vi "Unit test on Decode response.vi"() -> (0 "Error array":errorcluster[](array[cluster]), 2 "Test results":T1(array[cluster]), 3 "Passed":bool)   [LabVIEW 2021, in "F-70 driver.lvlib"]
uses:
  F-70 driver.lvlib
  public/F-70 parameters.ctl
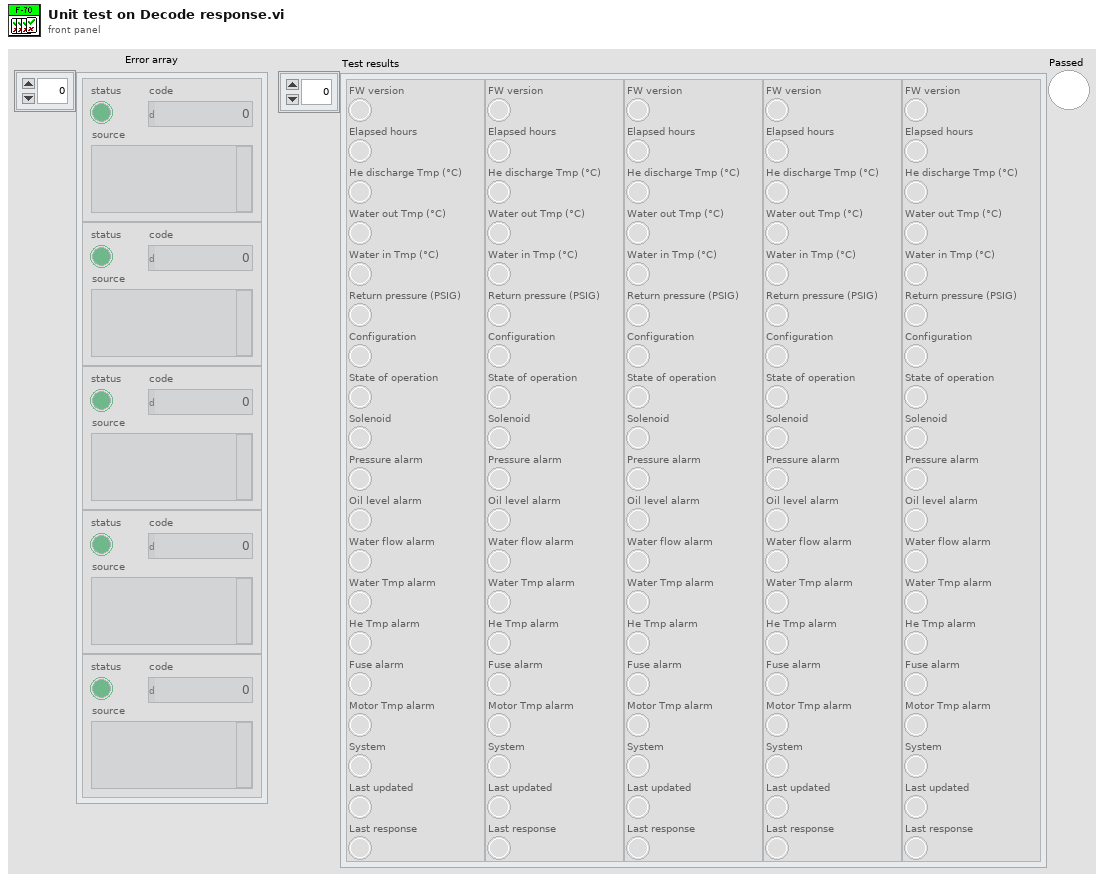
[diagram p1: front panel]
types:
  T1 = cluster{"FW version":bool, "Elapsed hours":bool, "He discharge Tmp (°C)":bool, "Water out Tmp (°C)":bool, "Water in Tmp (°C)":bool, "Return pressure (PSIG)":bool, "Configuration":bool, "State of operation":bool, "Solenoid":bool, "Pressure alarm":bool, "Oil level alarm":bool, "Water flow alarm":bool, "Water Tmp alarm":bool, "He Tmp alarm":bool, "Fuse alarm":bool, "Motor Tmp alarm":bool, "System":bool, "Last updated":bool, "Last response":bool}[]
  T2 = typedef "F-70 driver.lvlib/F-70 parameters.ctl" = cluster{"FW version":dbl, "Elapsed hours":dbl, "He discharge Tmp (°C)":dbl, "Water out Tmp (°C)":dbl, "Water in Tmp (°C)":dbl, "Return pressure (PSIG)":dbl, "Configuration":bool, "State of operation":u16, "Solenoid":bool, "Pressure alarm":bool, "Oil level alarm":bool, "Water flow alarm":bool, "Water Tmp alarm":bool, "He Tmp alarm":bool, "Fuse alarm":bool, "Motor Tmp alarm":bool, "System":bool, "Last updated":timestamp, "Last response":string}
  T3 = cluster{"FW version":bool, "Elapsed hours":bool, "He discharge Tmp (°C)":bool, "Water out Tmp (°C)":bool, "Water in Tmp (°C)":bool, "Return pressure (PSIG)":bool, "Configuration":bool, "State of operation":bool, "Solenoid":bool, "Pressure alarm":bool, "Oil level alarm":bool, "Water flow alarm":bool, "Water Tmp alarm":bool, "He Tmp alarm":bool, "Fuse alarm":bool, "Motor Tmp alarm":bool, "System":bool, "Last updated":bool, "Last response":bool}
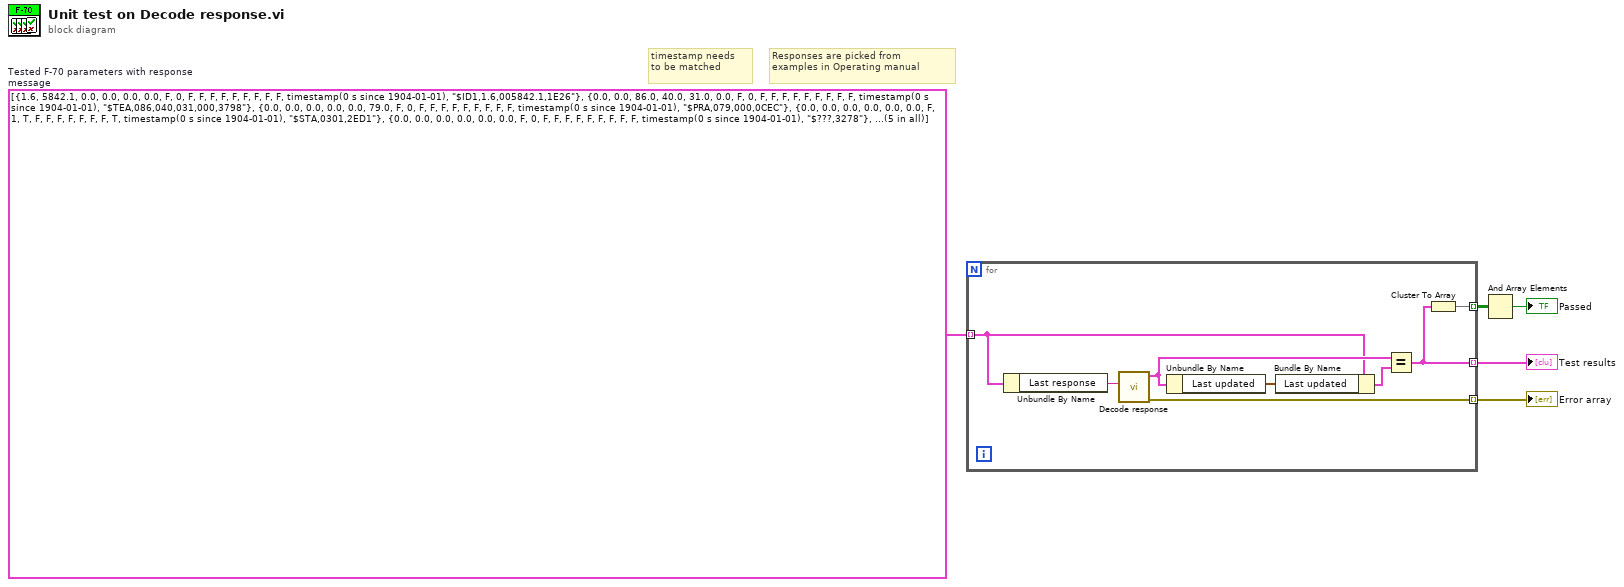
[diagram p0: block diagram]
diagram:
  w5 = T2[] [{"FW version"=1.6, "Elapsed hours"=5842.1, "He discharge Tmp (°C)"=0.0, "Water out Tmp (°C)"=0.0, "Water in Tmp (°C)"=0.0, "Return pressure (PSIG)"=0.0, "Configuration"=FALSE, "State of operation"=0, "Solenoid"=FALSE, "Pressure alarm"=FALSE, "Oil level alarm"=FALSE, "Water flow alarm"=FALSE, "Water Tmp alarm"=FALSE, "He Tmp alarm"=FALSE, "Fuse alarm"=FALSE, "Motor Tmp alarm"=FALSE, "System"=FALSE, "Last updated"=timestamp(0 s since 1904-01-01), "Last response"="$ID1,1.6,005842.1,1E26"}, {"FW version"=0.0, "Elapsed hours"=0.0, "He discharge Tmp (°C)"=86.0, "Water out Tmp (°C)"=40.0, "Water in Tmp (°C)"=31.0, "Return pressure (PSIG)"=0.0, "Configuration"=FALSE, "State of operation"=0, "Solenoid"=FALSE, "Pressure alarm"=FALSE, "Oil level alarm"=FALSE, "Water flow alarm"=FALSE, "Water Tmp alarm"=FALSE, "He Tmp alarm"=FALSE, "Fuse alarm"=FALSE, "Motor Tmp alarm"=FALSE, "System"=FALSE, "Last updated"=timestamp(0 s since 1904-01-01), "Last response"="$TEA,086,040,031,000,3798"}, {"FW version"=0.0, "Elapsed hours"=0.0, "He discharge Tmp (°C)"=0.0, "Water out Tmp (°C)"=0.0, "Water in Tmp (°C)"=0.0, "Return pressure (PSIG)"=79.0, "Configuration"=FALSE, "State of operation"=0, "Solenoid"=FALSE, "Pressure alarm"=FALSE, "Oil level alarm"=FALSE, "Water flow alarm"=FALSE, "Water Tmp alarm"=FALSE, "He Tmp alarm"=FALSE, "Fuse alarm"=FALSE, "Motor Tmp alarm"=FALSE, "System"=FALSE, "Last updated"=timestamp(0 s since 1904-01-01), "Last response"="$PRA,079,000,0CEC"}, {"FW version"=0.0, "Elapsed hours"=0.0, "He discharge Tmp (°C)"=0.0, "Water out Tmp (°C)"=0.0, "Water in Tmp (°C)"=0.0, "Return pressure (PSIG)"=0.0, "Configuration"=FALSE, "State of operation"=1, "Solenoid"=TRUE, "Pressure alarm"=FALSE, "Oil level alarm"=FALSE, "Water flow alarm"=FALSE, "Water Tmp alarm"=FALSE, "He Tmp alarm"=FALSE, "Fuse alarm"=FALSE, "Motor Tmp alarm"=FALSE, "System"=TRUE, "Last updated"=timestamp(0 s since 1904-01-01), "Last response"="$STA,0301,2ED1"}, {"FW version"=0.0, "Elapsed hours"=0.0, "He discharge Tmp (°C)"=0.0, "Water out Tmp (°C)"=0.0, "Water in Tmp (°C)"=0.0, "Return pressure (PSIG)"=0.0, "Configuration"=FALSE, "State of operation"=0, "Solenoid"=FALSE, "Pressure alarm"=FALSE, "Oil level alarm"=FALSE, "Water flow alarm"=FALSE, "Water Tmp alarm"=FALSE, "He Tmp alarm"=FALSE, "Fuse alarm"=FALSE, "Motor Tmp alarm"=FALSE, "System"=FALSE, "Last updated"=timestamp(0 s since 1904-01-01), "Last response"="$???,3278"}]  # Tested F-70 parameters with response message
  # "Responses are picked from \nexamples in Operating manual"
  # "timestamp needs\nto be matched"
  n1 = for {
    tunnel: w5 -> [w6] mode=indexing
    tunnel: [w13] -> w4 mode=indexing
    tunnel: [w11] -> w3 mode=indexing
    tunnel: [w10] -> w2 mode=indexing
    n2 = Unbundle By Name(w6) -> ("Last response"=w12:string)
    n3 = call "Decode response.vi"("response in"=w12) -> ("error out"=w13:errorcluster, "F-70 parameters out"=w7:T2)  [unwired: 9 in]
    n4 = Unbundle By Name(w7) -> ("Last updated"=w9:timestamp)
    n5 = Bundle By Name(cluster=w6, "Last updated"=w9) -> (w8:T2)
    n6 = Equal?(x=w7, y=w8) -> (x = y?=w11:T3)
    n7 = Cluster To Array(cluster=w11) -> (array=w10:bool[])
  }
  "Error array" <- w4
  "Test results" <- w3
  n8 = And Array Elements(Boolean array=w2) -> (logical AND=→"Passed":bool)
